vi "GetPosSingleAxis.vi"(8 "error in (no error)":errorcluster, 10 "Axis":i32=1 min=1 max=4, 11 "DelayLine in":refnum<class "DelayLine.lvclass">) -> (0 "error out":errorcluster, 2 "Pos":dbl, 3 "DelayLine out":refnum<class "DelayLine.lvclass">)   [LabVIEW 2018, in "DelayLine.lvclass"]
uses:
  DelayLine.lvclass
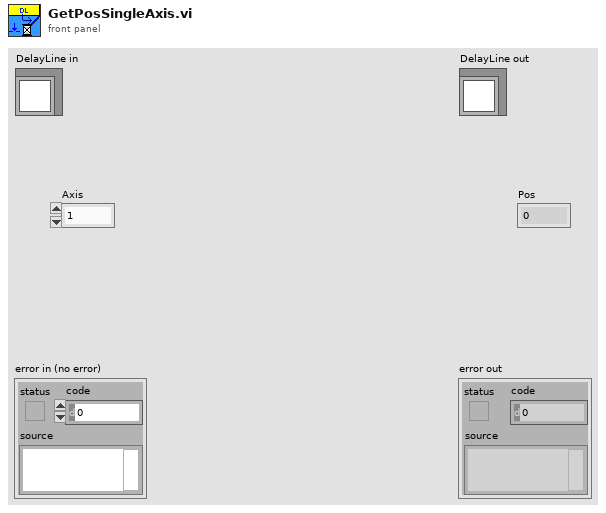
[diagram p1: front panel]
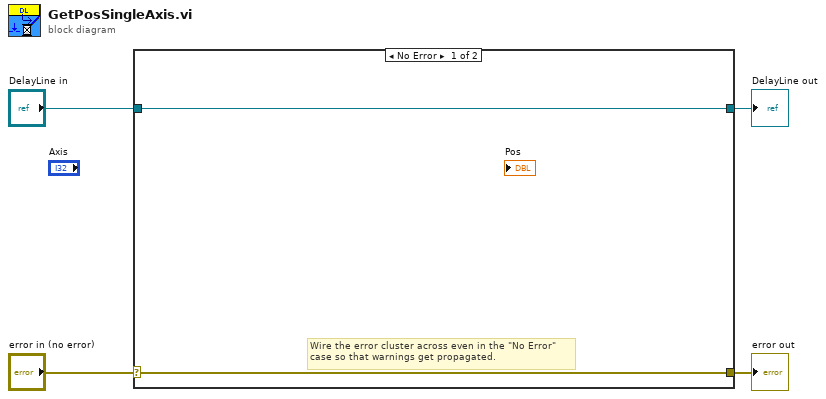
[diagram p0: block diagram]
diagram:
  n1 = case shown="No Error" "error in (no error)" {
    selector: "error in (no error)" -> [w5 w8]
    tunnel: [w5 w8] -> w3
    tunnel: [w6 w7] -> w1
    tunnel: "DelayLine in" -> [w6 w7]
    frame No Error {
      # "Wire the error cluster across even in the \"No Error\"\ncase so that warnings get propagated."
    }
    frame Error {
    }
  }
  "error out" <- w3
  "DelayLine out" <- w1
